vi "LV SciSDK FRAME.vi"(8 "error in (no error)":errorcluster, 9 "Frame Handle In":T2, 10 "Buffer Size":i32) -> (0 "error out":errorcluster, 1 "Frame Handle Out":T2, 2 "buffer out":T1)   [LabVIEW 2021]
uses:
  SciSDK_Labview.lvlib
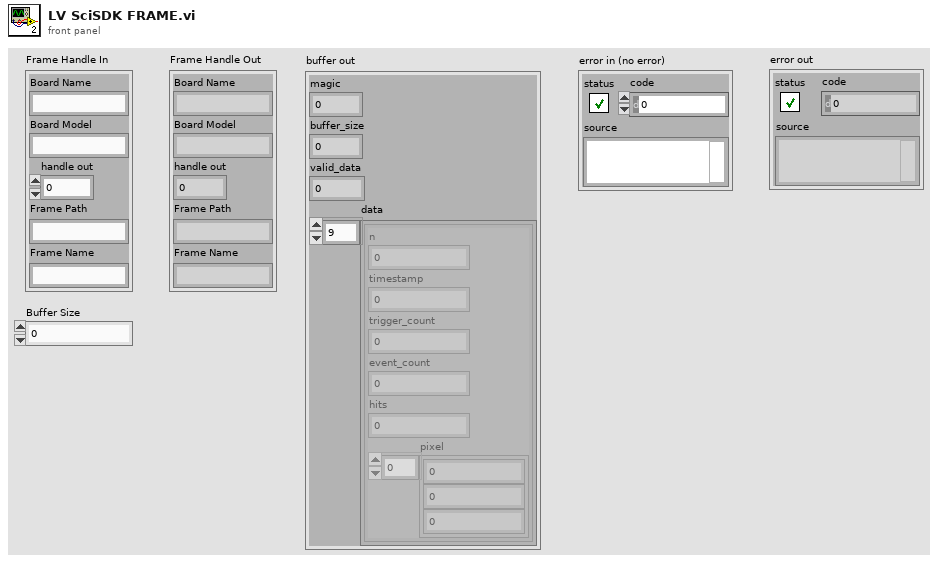
[diagram p1: front panel]
types:
  T1 = cluster{"magic":u32, "buffer_size":u32, "valid_data":u32, "data":cluster{"n":u64, "timestamp":u64, "trigger_count":u64, "event_count":u64, "hits":u64, "pixel":u32[]}[]}
  T2 = cluster{"Board Name":string, "Board Model":string, "handle out":u64, "Frame Path":string, "Frame Name":string}
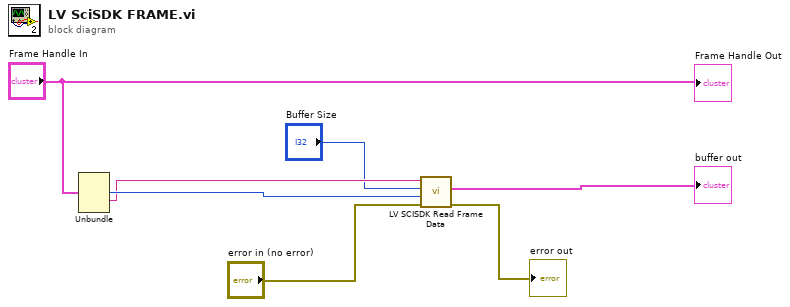
[diagram p0: block diagram]
diagram:
  n1 = Unbundle("Frame Handle In") -> ("handle out"=w6:u64, "Frame Path"=w5:string)  [unwired: 3 out]
  n2 = call "LV SCISDK Read Frame Data.vi"("Path"=w5, "buffer_size"="Buffer Size", "handle"=w6, "error in (no error)"="error in (no error)") -> ("buffer out"=→"buffer out":T1, "error out"=→"error out":errorcluster)  [unwired: 3 in, 2 out]
  "Frame Handle Out" <- "Frame Handle In"
